vi "Untitled 11.vi"() -> ()   [LabVIEW 2011]
panel:
  out "x = y?":bool
  out "NaN/Path/Refnum? 2":bool
  out "NaN/Path/Refnum?":bool
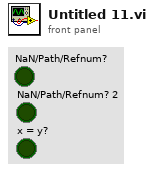
[diagram p1: front panel]
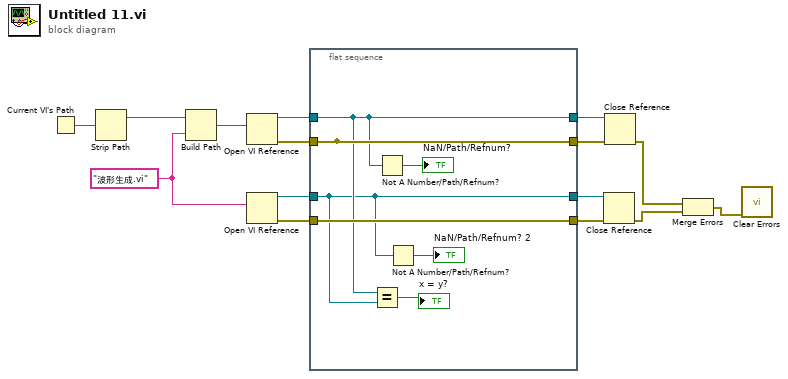
[diagram p0: block diagram]
diagram:
  w12 = "波形生成.vi" ("name or relative path")
  n1 = Current VI's Path() -> (path=w15:path)
  n2 = Strip Path(path=w15) -> (stripped path=w14:path)  [unwired: 1 out]
  n3 = Build Path(base path=w14, name or relative path=w12) -> (appended path=w13:path)
  n4 = Open VI Reference(vi path=w13) -> (vi reference=w11:refnum<vi>, error out=w10:errorcluster)  [unwired: 5 in]
  n5 = Open VI Reference(vi path=w12) -> (vi reference=w9:refnum<vi>, error out=w8:errorcluster)  [unwired: 5 in]
  n6 = flat-sequence {
    tunnel: w11 -> [w19]
    tunnel: w10 -> [w21]
    tunnel: w9 -> [w18]
    tunnel: w8 -> [w22]
    tunnel: [w19] -> w7
    tunnel: [w21] -> _
    tunnel: [w18] -> w5
    tunnel: [w22] -> w4
    tunnel: [w21] -> w6
    frame #0 {
      n7 = Equal?(x=w19, y=w18) -> (x = y?=→"x = y?":bool)
      n8 = Not A Number/Path/Refnum?(number/path/refnum=w19) -> (NaN/Path/Refnum?=→"NaN/Path/Refnum?":bool)
      n9 = Not A Number/Path/Refnum?(number/path/refnum=w18) -> (NaN/Path/Refnum?=→"NaN/Path/Refnum? 2":bool)
    }
  }
  n10 = Close Reference(reference=w5, error in (no error)=w4) -> (error out=w2:errorcluster)
  n11 = Close Reference(reference=w7, error in (no error)=w6) -> (error out=w3:errorcluster)
  n12 = Merge Errors(w3, w2) -> (w1:errorcluster)
  n13 = call <vilib>:"Clear Errors.vi"("error in (no error)"=w1) -> ()  [unwired: 6 in, 1 out]
